vi "Init.vi"(8 "error in (no error)":errorcluster, 10 "ID":string, 11 "Channel in":refnum<class "Channel.lvclass">) -> (0 "error out":errorcluster, 3 "Channel out":refnum<class "Channel.lvclass">)   [LabVIEW 2020, in "Channel.lvclass"]
uses:
  Channel.lvclass
  Packed Libraries/Audio Processing.lvlibp/Value Cluster.ctl
  Packed Libraries/Audio Processing.lvlibp/Value Properties.ctl
  EQ.ctl
  Channel.lvclass/Channel.ctl
  Packed Libraries/Messaging.lvlibp
  Packed Libraries/Audio Processing.lvlibp
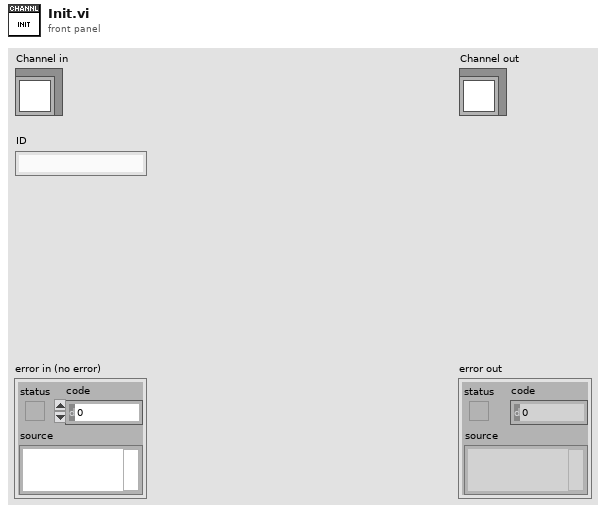
[diagram p1: front panel]
types:
  T1 = typedef "Audio Processing.lvlibp/Value Cluster.ctl" = cluster{"Value":dbl, "Properties":T2}
  T2 = typedef "Audio Processing.lvlibp/Value Properties.ctl" = cluster{"Lower":dbl, "Upper":dbl, "Default":dbl, "Increment":dbl}
  T3 = typedef "Channel.lvclass/EQ.ctl" = cluster{"Level":T1, "Kill":bool}
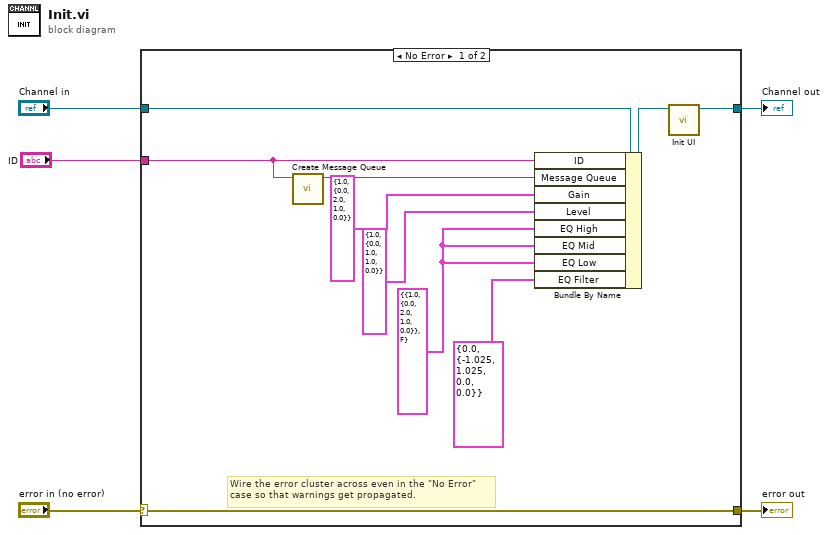
[diagram p0: block diagram]
diagram:
  n1 = case shown="No Error" "error in (no error)" {
    selector: "error in (no error)" -> [w15 w17]
    tunnel: [w15 w17] -> w4
    tunnel: [w6 w16] -> w2
    tunnel: "Channel in" -> [w14 w16]
    tunnel: "ID" -> [w13 _]
    frame No Error {
      w11 = T3 {"Level"={"Value"=1.0, "Properties"={"Lower"=0.0, "Upper"=2.0, "Default"=1.0, "Increment"=0.0}}, "Kill"=FALSE} ("EQ High")
      # "Wire the error cluster across even in the \"No Error\"\ncase so that warnings get propagated."
      n2 = call "Create Message Queue.vi"("Queue Name"=w13) -> ("queue out"=w12:refnum<queue>)  [unwired: 9 in, 1 out]
      n3 = Bundle By Name(cluster=w14, "ID"=w13, "Message Queue"=w12, "Gain"=T1 {"Value"=1.0, "Properties"={"Lower"=0.0, "Upper"=2.0, "Default"=1.0, "Increment"=0.0}} ("Level"), "Level"=T1 {"Value"=1.0, "Properties"={"Lower"=0.0, "Upper"=1.0, "Default"=1.0, "Increment"=0.0}}, "EQ High"=w11, "EQ Mid"=w11, "EQ Low"=w11, "EQ Filter"=T1 {"Value"=0.0, "Properties"={"Lower"=-1.025, "Upper"=1.025, "Default"=0.0, "Increment"=0.0}} ("Level")) -> (w7:refnum<class "Channel.lvclass">)
      n4 = call "Init UI.vi"("Channel in"=w7) -> ("Channel out"=w6:refnum<class "Channel.lvclass">)  [unwired: 9 in, 1 out]
    }
    frame Error {
    }
  }
  "error out" <- w4
  "Channel out" <- w2
